vi "frontsB.vi"(3 "IN":bool[](array[boolean])) -> (0 "FALL":bool[](array[boolean]), 1 "RAISE":bool[](array[boolean]))   [LabVIEW 2019, in "Logik.lvlib"]
uses:
  Logik.lvlib
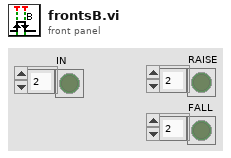
[diagram p1: front panel]
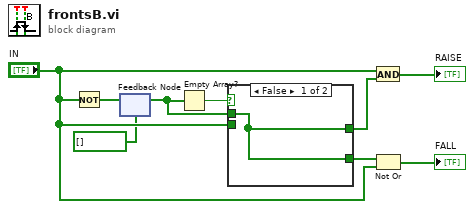
[diagram p0: block diagram]
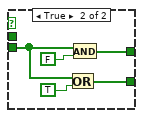
[diagram p2: hidden frame]
diagram:
  n1 = Not(x="IN") -> (.not. x?=w7:bool[])
  n2 = feedback #1(bool[] []) -> (w5:bool[])
  n3 = feedback-in #1(w7) -> ()
  n4 = Empty Array?(array=w5) -> (empty?=w4:bool)
  n5 = case shown="False" w4 {
    tunnel: "IN" -> [_ w11]
    tunnel: w5 -> [w10 _]
    tunnel: [w10 w13] -> w2
    tunnel: [w10 w12] -> w3
    frame False {
    }
    frame True {
      n6 = Or(x=w11, y=TRUE ("IN")) -> (x .or. y?=w12:bool[])
      n7 = And(x=w11, y=FALSE ("IN")) -> (x .and. y?=w13:bool[])
    }
  }
  n8 = And(x="IN", y=w2) -> (x .and. y?=→"RAISE":bool[])
  n9 = Not Or(1:"IN", 2:w3) -> (0:→"FALL":bool[])
